vi "determine_N_v07.vi"(0 "Pulse Data in (pA)":waveform(dbl)[](graph), 1 "memtest":T2={"Samples to Read"=2000, "Rate (Hz)"=20000.0, "Amplitude (mV/pA)"=10.0, "Offset (mV/pA)"=0.0, "Frequency (Hz)"=10.0, "duty cycle (%)"=50.0, "phase"=0.0} {"phase" format="%.2p"; "duty cycle (%)" format="%0.2f"}, 2 "replicates":i32=5, 3 "error in":errorcluster, 4 "Noise Data in (pA)":waveform(dbl)[](graph)) -> (5 "Waveform Graph":waveform(dbl)[](graph), 6 "Power Spectrum":dbl[](graph), 7 "avg peak height":dbl, 8 "cell quality bad":bool, 9 "cell stats":T1 {"STD" format="%010.2f"; "Variance" format="%010.2f"; "Rt (MOhms)" format="%010.2f"; "tau (ms)" format="%08.2g"; "Cm (pF)" format="%08.2f"; "Ra (MOhms)" format="%010.2f"; "Rm (MOhms)" format="%010.2f"; "Ihold (pA)" format="%010.2f"}, 10 "error out":errorcluster)   [LabVIEW 2015]
uses:
  wc_protocol_v1.003 Folder/whole_cell_protocol/Controls/cell_stats-v02.ctl
  <vilib>/Analysis/NI_AALPro.lvlib
  <vilib>/Analysis/2dsp.llb/Power Spectrum (DBL).vi
  controls/memtest_def.ctl
panel:
  out "Variance":dbl
  out "STD":dbl
  out "C (pF)":dbl
  out "Q (pA * s)":dbl format="%0.4f"
  out "transient":dbl[](graph)
  in  "fraction for Q":dbl=0.05
  out "t_stimOn":dbl
  out "Rm (MOhms)":dbl
  out "Ra (MOhms)":dbl
  out "peak value (pA)":dbl
  out "peak time (samples)":i32
  in  "peakOffset (samples)":i32=2
  out "first mean":dbl format="%0.2f"
  out "duration 2":dbl
  out "t_startFirst":dbl
  out "t_startSecond":dbl
  out "duration 1":dbl
  out "t_stimOff":dbl
  in  "fractionToSample":dbl=0.1
  out "R_total (MOhms)":dbl format="%#_13g"
  out "holding current out (pA)":dbl format="%#_13g"
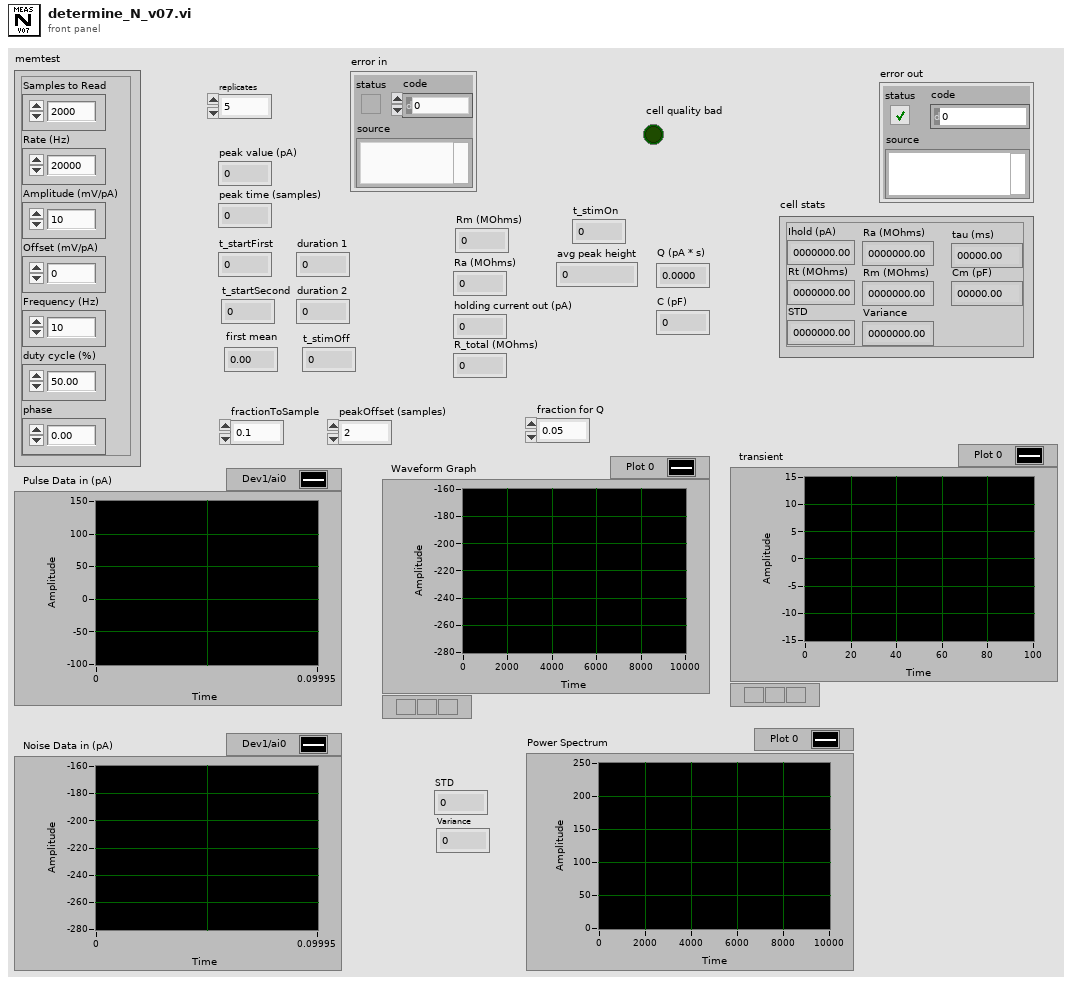
[diagram p1: front panel]
types:
  T1 = typedef "cell_stats-v02.ctl" = cluster{"Ihold (pA)":dbl, "Rm (MOhms)":dbl, "Ra (MOhms)":dbl, "Cm (pF)":dbl, "tau (ms)":dbl, "Rt (MOhms)":dbl, "Variance":dbl, "STD":dbl}
  T2 = typedef "memtest_def.ctl" = cluster{"Samples to Read":i32, "Rate (Hz)":dbl, "Amplitude (mV/pA)":dbl, "Offset (mV/pA)":dbl, "Frequency (Hz)":dbl, "duty cycle (%)":dbl, "phase":dbl}
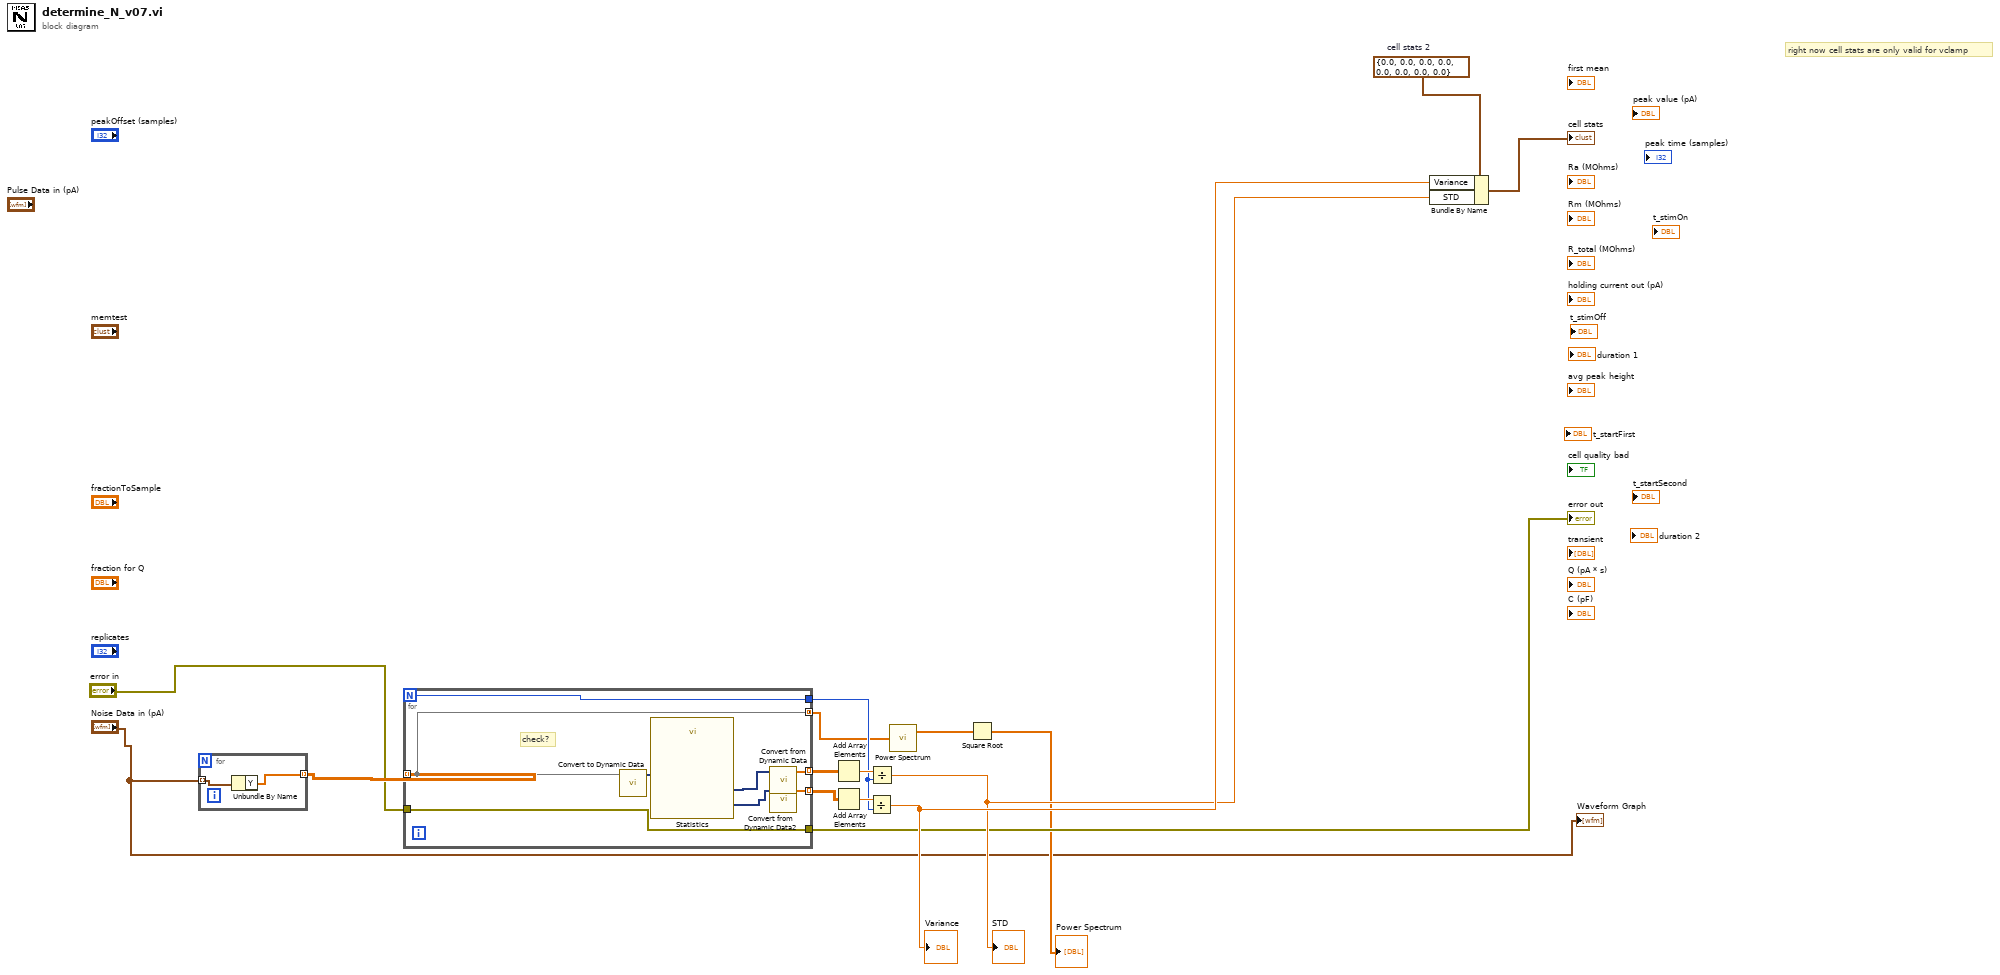
[diagram p0: block diagram]
diagram:
  w11 = T1 {"Ihold (pA)"=0.0, "Rm (MOhms)"=0.0, "Ra (MOhms)"=0.0, "Cm (pF)"=0.0, "tau (ms)"=0.0, "Rt (MOhms)"=0.0, "Variance"=0.0, "STD"=0.0}  # cell stats 2
  # "right now cell stats are only valid for vclamp"
  n1 = for {
    tunnel: "Noise Data in (pA)" -> [w18] mode=indexing
    tunnel: [w17] -> w15 mode=indexing
    n2 = Unbundle By Name(w18) -> ("Y"=w17:dbl[])
  }
  n3 = for {
    N -> [w25]
    tunnel: w15 -> [w20] mode=indexing
    tunnel: [w25] -> w6
    tunnel: [w20] -> w2 mode=concatenating
    tunnel: [w23] -> w10 mode=indexing
    tunnel: [w21] -> w9 mode=indexing
    tunnel: "error in" -> [w19]
    tunnel: [w19] -> w4
    # "check?"
    n4 = call "Convert to Dynamic Data"("Array"=w20) -> ("Dynamic Data Type"=w26:dynamicdata)  [unwired: 3 in]
    n5 = call "Statistics"("Signals"=w26) -> ("Variance"=w22:dynamicdata, "Standard Dev"=w24:dynamicdata)  [unwired: 24 in, 1 out]
    n6 = call "Convert from Dynamic Data"("Dynamic Data Type"=w24) -> ("Array"=w23:dbl[])  [unwired: 3 in]
    n7 = call "Convert from Dynamic Data2"("Dynamic Data Type"=w22) -> ("Array"=w21:dbl[])  [unwired: 3 in]
  }
  "error out" <- w4
  n8 = Add Array Elements(numeric array=w10) -> (sum=w8:dbl)
  n9 = Add Array Elements(numeric array=w9) -> (sum=w7:dbl)
  n10 = Divide(x=w7, y=w6) -> (x/y=w13:dbl)
  "Variance" <- w13
  n11 = Divide(x=w8, y=w6) -> (x/y=w12:dbl)
  "STD" <- w12
  n12 = call-poly <vilib>:"Power Spectrum.vi"("X"=w2) -> ("Power Spectrum"=w14:dbl[])  [unwired: 1 out]
  n13 = Square Root(x=w14) -> (sqrt(x)=→"Power Spectrum":dbl[])
  n14 = Bundle By Name(cluster=w11, "Variance"=w13, "STD"=w12) -> (→"cell stats":T1)
  "Waveform Graph" <- "Noise Data in (pA)"
